vi "add_freq_char_to_report.vi"(8 "error in (no error)":errorcluster, 11 "Boc12 in":refnum<class "Boc12.lvclass">) -> (0 "error out":errorcluster, 3 "Boc12 out":refnum<class "Boc12.lvclass">)   [LabVIEW 2017, in "Boc12.lvclass"]
uses:
  Boc12.lvclass
  Report.lvclass/Report.ctl
  <vilib>/Utility/NIReport.llb/Append Text Table to Report (wrap).vi
  <vilib>/Utility/NIReport.llb/NI_report.lvclass
  Report.lvclass
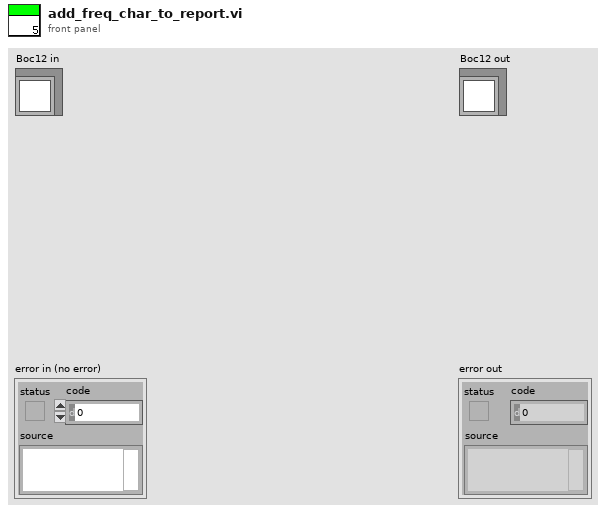
[diagram p1: front panel]
types:
  T1 = cluster{"position (excel)":cluster{"row":i32, "column":i32}, "name (excel)":string, "bookmark (word)":string}
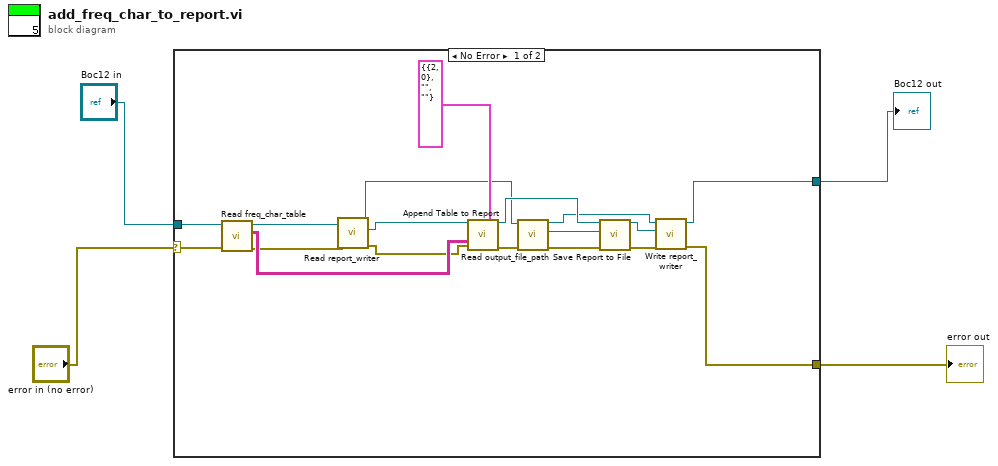
[diagram p0: block diagram]
diagram:
  n1 = case shown="No Error" "error in (no error)" {
    selector: "error in (no error)" -> [w18 w23]
    tunnel: [w9 w23] -> w3
    tunnel: [w8 w24] -> w2
    tunnel: "Boc12 in" -> [w19 w24]
    frame No Error {
      n2 = call-dynamic "Read freq_char_table.vi"("error in (no error)"=w18, "Report in"=w19) -> ("error out"=w17:errorcluster, "freq_char_table"=w20:string[][], "Report out"=w16:refnum<class "Boc12.lvclass">)  [unwired: 7 in]
      n3 = call "Read report_writer.vi"("error in (no error)"=w17, "Report in"=w16) -> ("error out"=w14:errorcluster, "NI_report.lvclass"=w15:refnum<class "NI_report.lvclass">, "Report out"=w11:refnum<class "Boc12.lvclass">)  [unwired: 7 in]
      n4 = call-poly <vilib>:"Append Table to Report.vi"("report in"=w15, "MS Office parameters"=T1 {"position (excel)"={"row"=2, "column"=0}, "name (excel)"="", "bookmark (word)"=""}, "text data"=w20, "error in (no error)"=w14) -> ("report out"=w21:refnum<class "NI_report.lvclass">, "error out"=w12:errorcluster)  [unwired: 8 in, 2 out]
      n5 = call "Read output_file_path.vi"("error in (no error)"=w12, "Report in"=w11) -> ("error out"=w13:errorcluster, "output_file_path"=w5:path, "Report out"=w6:refnum<class "Boc12.lvclass">)  [unwired: 7 in]
      n6 = call-dynamic "Save Report to File.vi"("report in"=w21, "report file path"=w5, "error in (no error)"=w13) -> ("report out"=w7:refnum<class "NI_report.lvclass">, "error out"=w10:errorcluster)  [unwired: 11 in]
      n7 = call "Write report_writer.vi"("error in (no error)"=w10, "NI_report.lvclass"=w7, "Report in"=w6) -> ("error out"=w9:errorcluster, "Report out"=w8:refnum<class "Boc12.lvclass">)  [unwired: 7 in]
    }
    frame Error {
    }
  }
  "error out" <- w3
  "Boc12 out" <- w2
